vi "Write Result.vi"(0 "Charact Result Accessor in":refnum<class "Result Accessor.lvclass">, 5 "Charact Result":variant, 11 "error in":errorcluster) -> (4 "Charact Result Accessor out":refnum<class "Result Accessor.lvclass">, 15 "error out":errorcluster)   [LabVIEW 2023, in "RFCalAndFixtureCharact.Common.lvlib" / "Result Accessor.lvclass"]
uses:
  Result Accessor.lvclass
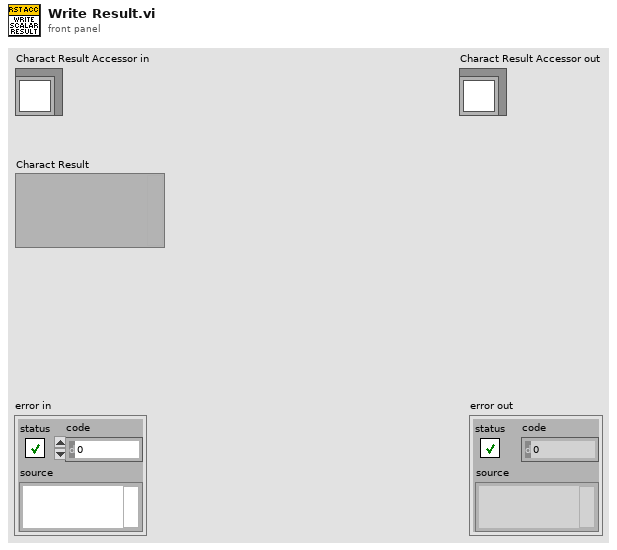
[diagram p1: front panel]
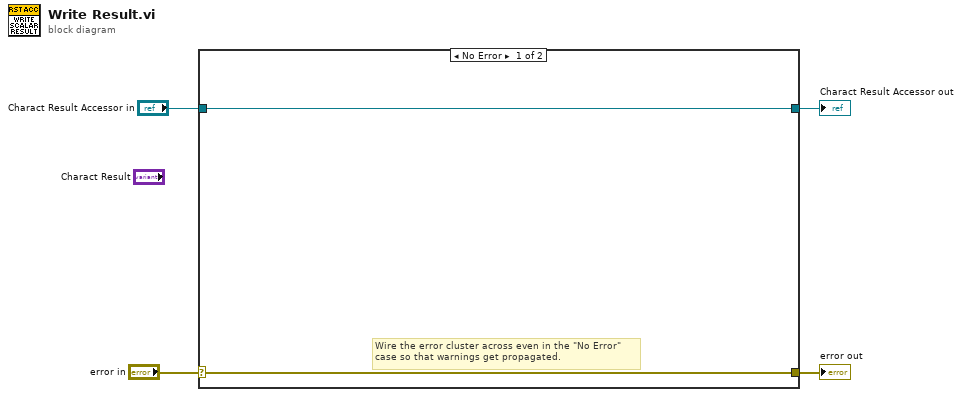
[diagram p0: block diagram]
diagram:
  n1 = case shown="No Error" "error in" {
    selector: "error in" -> [w5 w8]
    tunnel: [w5 w8] -> w3
    tunnel: [w6 w7] -> w1
    tunnel: "Charact Result Accessor in" -> [w6 w7]
    frame No Error {
      # "Wire the error cluster across even in the \"No Error\"\ncase so that warnings get propagated."
    }
    frame Error {
    }
  }
  "error out" <- w3
  "Charact Result Accessor out" <- w1
